vi "FaultAck.vi"   [LabVIEW 2019]
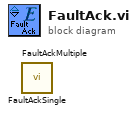
[diagram p0: block diagram]
diagram:
  n1 = call "FaultAckMultiple.vi"() -> ()  [unwired: 10 in, 2 out]
  n2 = call "FaultAckSingle.vi"() -> ()  [unwired: 10 in, 2 out]
